vi "ReadSV.vi"(8 "error in (no error)":errorcluster, 11 "shared variable refnum in":refnum<k21>) -> (0 "error out":errorcluster, 2 "DBL Data":dbl)   [LabVIEW 2016, in "Shared Variable Interface.lvlib" / "Bool.lvlib"]
uses:
  Bool.lvlib
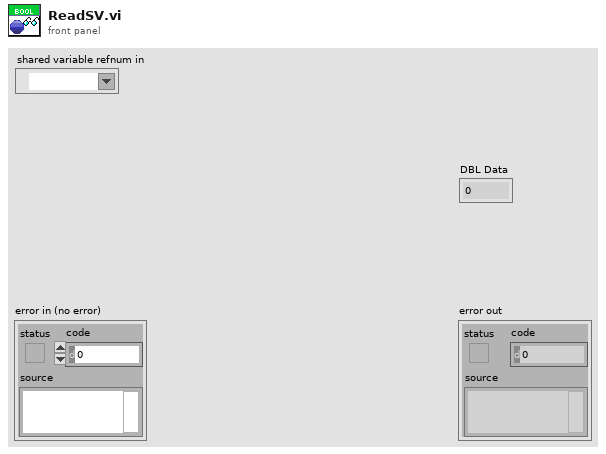
[diagram p1: front panel]
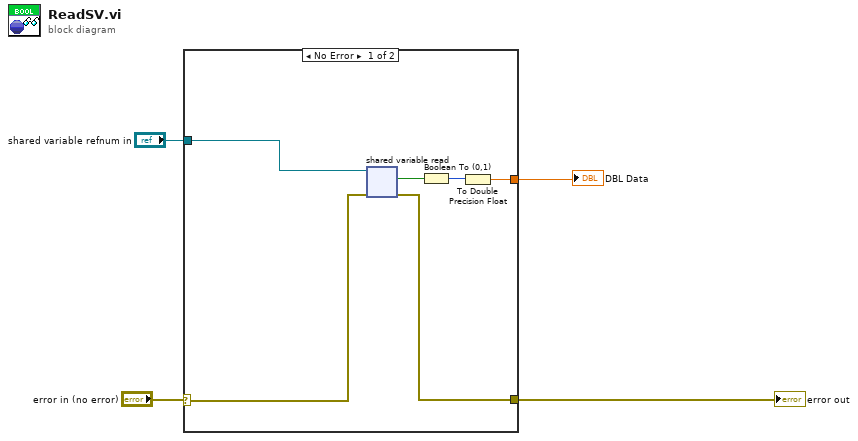
[diagram p0: block diagram]
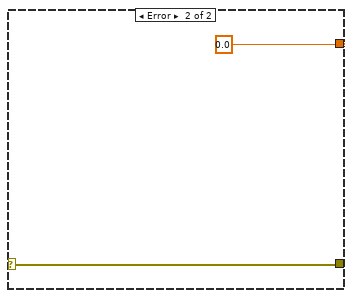
[diagram p2: hidden frame]
diagram:
  n1 = case shown="No Error" "error in (no error)" {
    selector: "error in (no error)" -> [w6 w12]
    tunnel: [w10 w12] -> w3
    tunnel: [w7 0.0] -> w2
    tunnel: "shared variable refnum in" -> [w5 _]
    frame No Error {
      n2 = shared-variable-read(w5, w6) -> (w10:errorcluster, w9:bool)  [unwired: 2 out]
      n3 = Boolean To (0,1)(Boolean=w9) -> (0, 1=w8:i16)
      n4 = To Double Precision Float(number=w8) -> (double precision float=w7:dbl)
    }
    frame Error {
    }
  }
  "error out" <- w3
  "DBL Data" <- w2
